vi "Untitled 2 (SubVI).vi"(6 "Y":dbl, 9 "X":dbl, 10 "Y 2":dbl[](array[numeric]), 11 "X 2":dbl[](array[numeric])) -> (2 "Array":dbl[](array[numeric]), 3 "Array 2":dbl[](array[numeric]))   [LabVIEW 2015]
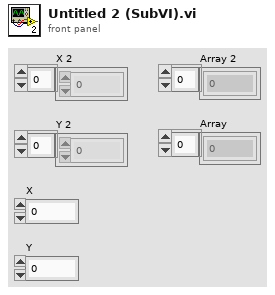
[diagram p1: front panel]
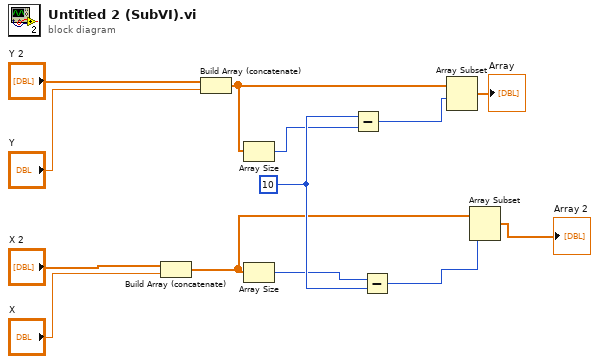
[diagram p0: block diagram]
diagram:
  w12 = 10
  n1 = Build Array (concatenate)("X 2", "X") -> (w7:dbl[])
  n2 = Build Array (concatenate)("Y 2", "Y") -> (w6:dbl[])
  n3 = Array Size(array=w6) -> (size(s)=w9:i32)
  n4 = Array Size(array=w7) -> (size(s)=w8:i32)
  n5 = Subtract(x=w12, y=w9) -> (x-y=w11:i32)
  n6 = Subtract(x=w8, y=w12) -> (x-y=w10:i32)
  n7 = Array Subset(array=w6, index=w11) -> (→"Array":dbl[])  [unwired: 1 in]
  n8 = Array Subset(array=w7, index=w10) -> (→"Array 2":dbl[])  [unwired: 1 in]
